vi "FTW-ERR-NoErrorConstant.vi"() -> (0 "no error":errorcluster)   [LabVIEW 2012]
panel:
  # "Outputs"
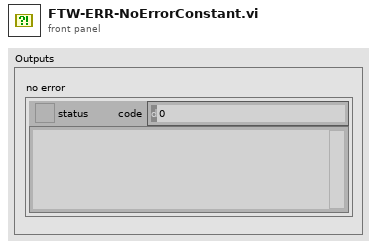
[diagram p1: front panel]
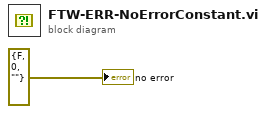
[diagram p0: block diagram]
diagram:
  "no error" <- errorcluster {"status"=FALSE, "code"=0, "source"=""} ("no error")
